vi "New Milan Box.vi"() -> ()   [LabVIEW 2019]
uses:
  Program Files (x86)/National Instruments/LabVIEW 2019/project/EN1Course-master (12)/EN1Course-master/_Subs/ThingWorx/_TW_Subs/TW_XControl.xctl
  <vilib>/httpClient/POSTBuffer.vi
  Program Files (x86)/National Instruments/LabVIEW 2019/project/EN1Course-master (12)/EN1Course-master/_Subs/ThingWorx/_TW_Subs/Thingworx_Write_string.vi
  <vilib>/httpClient/LabVIEWHTTPClient.lvlib
panel:
  in  "summary":string(xcontrol)
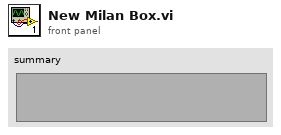
[diagram p1: front panel]
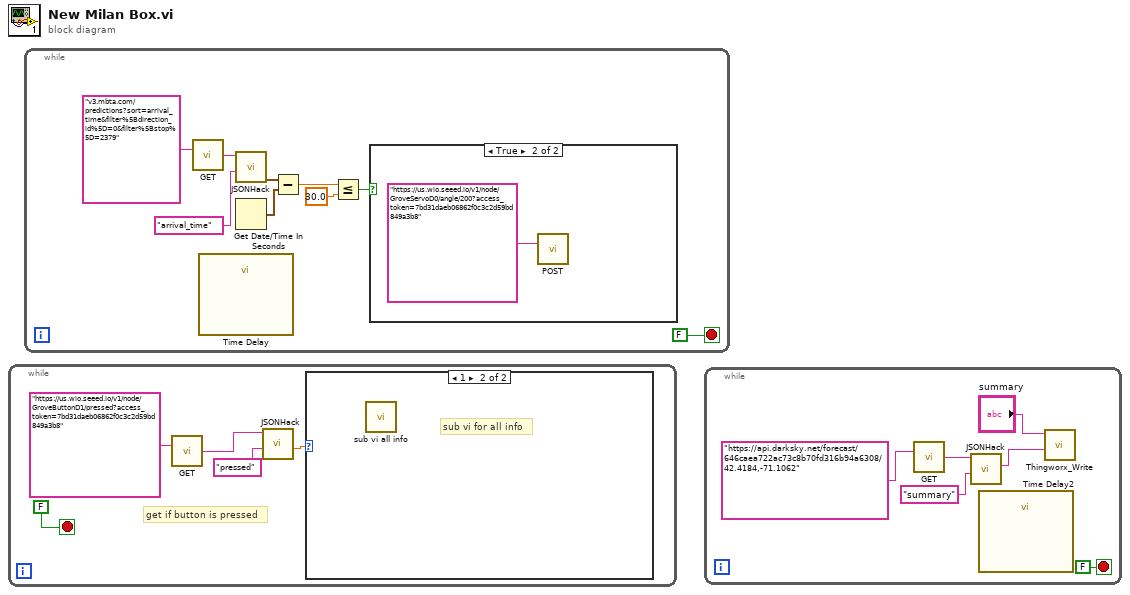
[diagram p0: block diagram]
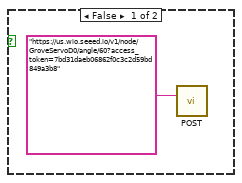
[diagram p2: hidden frame]
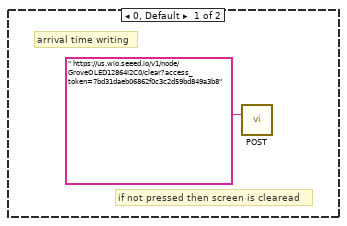
[diagram p3: hidden frame]
diagram:
  n1 = while {
    stop <- FALSE stop-if-true
    # "get if button is pressed"
    n2 = call <vilib>:"GET.vi"("url"="https://us.wio.seeed.io/v1/node/GroveButtonD1/pressed?access_token=7bd31daeb06862f0c3c2d59bd849a3b8") -> ("body"=w4:string)  [unwired: 11 in, 3 out]
    n3 = call "JSONHack.vi"("search name"="pressed", "JSON in"=w4) -> ("Property (num)"=w3:dbl)  [unwired: 6 in, 3 out]
    n4 = case shown="1" w3 {
      frame 0, Default {
        # "arrival time writing"
        # "if not pressed then screen is clearead"
        n5 = call-poly <vilib>:"POST.vi"("url"=" https://us.wio.seeed.io/v1/node/GroveOLED12864I2C0/clear?access_token=7bd31daeb06862f0c3c2d59bd849a3b8") -> ()  [unwired: 11 in, 4 out]
      }
      frame 1 {
        # "sub vi for all info"
        n6 = call "sub vi all info.vi"() -> ()  [unwired: 12 in]
      }
    }
  }
  n7 = while {
    stop <- FALSE stop-if-true
    n8 = call <vilib>:"GET.vi"("url"="v3.mbta.com/predictions?sort=arrival_time&filter%5Bdirection_id%5D=0&filter%5Bstop%5D=2379") -> ("body"=w15:string)  [unwired: 11 in, 3 out]
    n9 = call "Time Delay"() -> ()  [unwired: 11 in, 1 out]
    n10 = call "JSONHack.vi"("search name"="arrival_time", "JSON in"=w15) -> ("Property (time stamp)"=w12:timestamp)  [unwired: 6 in, 3 out]
    n11 = Get Date/Time In Seconds() -> (seconds since 1Jan1904=w11:timestamp)
    n12 = Subtract(x=w12, y=w11) -> (x-y=w10:dbl)
    n13 = Less Or Equal?(x=w10, y=30.0) -> (x <= y?=w8:bool)
    n14 = case shown="True" w8 {
      frame False {
        n15 = call-poly <vilib>:"POST.vi"("url"="https://us.wio.seeed.io/v1/node/GroveServoD0/angle/60?access_token=7bd31daeb06862f0c3c2d59bd849a3b8") -> ()  [unwired: 11 in, 4 out]
      }
      frame True {
        n16 = call-poly <vilib>:"POST.vi"("url"="https://us.wio.seeed.io/v1/node/GroveServoD0/angle/200?access_token=7bd31daeb06862f0c3c2d59bd849a3b8") -> ()  [unwired: 11 in, 4 out]
      }
    }
  }
  n17 = while {
    stop <- FALSE stop-if-true
    n18 = call <vilib>:"GET.vi"("url"="https://api.darksky.net/forecast/646caea722ac73c8b70fd316b94a6308/42.4184,-71.1062") -> ("body"=w22:string)  [unwired: 11 in, 3 out]
    n19 = call "JSONHack.vi"("search name"="summary", "JSON in"=w22) -> ("Property (str)"=w20:string)  [unwired: 6 in, 3 out]
    n20 = call "Time Delay2"() -> ()  [unwired: 11 in, 1 out]
    n21 = call-poly "Thingworx_Write.vi"("String"=w20, "Thingworx"="summary") -> ()  [unwired: 10 in]
  }
